vi "random_U16.vi"(1 "Offset":u16, 2 "Range":u16) -> (0 "Out":u16)   [LabVIEW 2013]
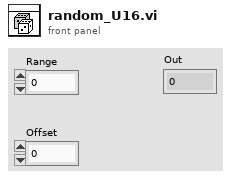
[diagram p1: front panel]
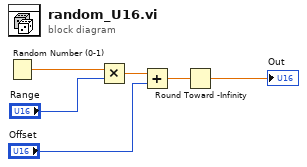
[diagram p0: block diagram]
diagram:
  n1 = Random Number (0-1)() -> (number: 0 to 1=w5:dbl)
  n2 = Multiply(x=w5, y="Range") -> (x*y=w3:dbl)
  n3 = Add(x=w3, y="Offset") -> (x+y=w2:dbl)
  n4 = Round Toward -Infinity(1:w2) -> (0:→"Out":dbl)
